vi "copy_packed_data.vi"(3 "error in":errorcluster, 5 "p":u64) -> (0 "error out":errorcluster, 1 "data":string, 2 "p out":u64)   [LabVIEW 2019, in "msgpack.lvlib"]
doc: "Copies the current contents of the msgpack buffer into labview memory, returning it as a byte buffer (U8 array)"
uses:
  msgpack.lvlib
  msgpackalt.dll
panel:
  # "msgpack"
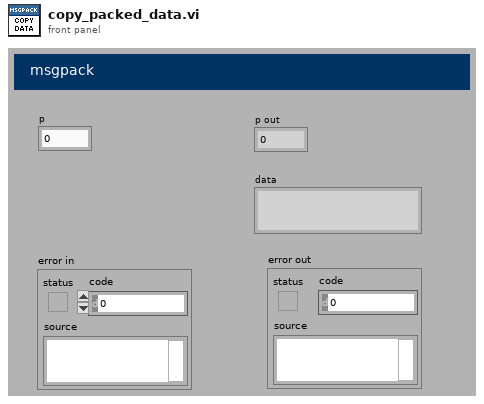
[diagram p1: front panel]
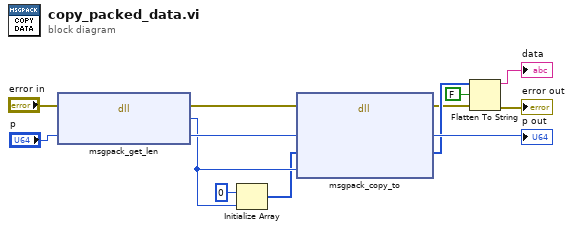
[diagram p0: block diagram]
diagram:
  n1 = dll-call lib="C:/Users/Patrick/Documents/GitHub/Instrument-Framework/lvsrc/SMOs/JSON-RPC-2019/lv-venv/lv.lib/vi.lib/addons/msgpack/msgpackalt.dll" fn="msgpack_get_len"(error in="error in", "p"="p") -> (error out=w9:errorcluster, "return type"=w8:u32, "p"=w11:u64)  [unwired: 2 in, 1 out]
  n2 = Initialize Array(u8 0 ("element"), w8) -> (w6:u8[])
  n3 = dll-call lib="C:/Users/Patrick/Documents/GitHub/Instrument-Framework/lvsrc/SMOs/JSON-RPC-2019/lv-venv/lv.lib/vi.lib/addons/msgpack/msgpackalt.dll" fn="msgpack_copy_to"(error in=w9, "p"=w11, "buffer"=w6, "max"=w8) -> (error out=w4:errorcluster, "p"=→"p out":u64, "buffer"=w5:u8[])  [unwired: 4 in, 1 out]
  n4 = Flatten To String(anything=w5, prepend array or string size? (T)=FALSE, error in (no error)=w4) -> (data string=→"data":string, error out=→"error out":errorcluster)  [unwired: 1 in, 1 out]
